vi "FPGANic.Globals.vi"() -> ()   [LabVIEW 2017]
panel:
  in  "IPv4 Message Counter":i16
  out "FPGA VI Reference Out":refnum<k20>
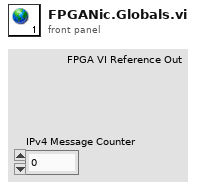
[diagram p1: front panel]
diagram:
